vi "Get Tx Generic Raw Frame List.vi"(8 "error in":errorcluster, 11 "custom device ref in":T3 format="%.0x") -> (0 "error out":errorcluster, 2 "Raw Frame List":T1[](array[typedef]) {"Data" format="%.0x"; "HeaderInfo"."NetSelect" items=["FDX_TX_FRAME_DLY_A"=0, "FDX_TX_FRAME_DLY_B"=1, "FDX_TX_FRAME_BOTH "=3, "FDX_TX_FRAME_ONLY_A"=4, "FDX_TX_FRAME_ONLY_B "=5]; "HeaderInfo"."FrameStartMode" items=["FDX_TX_FRAME_START_IFG", "FDX_TX_FRAME_START_PGWT", "FDX_TX_FRAME_START_TRG"]; "HeaderInfo"."PhysErrorInjection" items=["FDX_TX_FRAME_ERR_OFF"=0, "FDX_TX_FRAME_ERR_CRC"=1, "FDX_TX_FRAME_ERR_ALI"=2, "FDX_TX_FRAME_ERR_PRE"=4, "FDX_TX_FRAME_ERR_PHY"=8]; "HeaderInfo"."SequenceNumberInit" items=["FDX_TX_FRAME_SEQ_INIT_AUTO"=65535]; "HeaderInfo"."SequenceNumberOffset" items=["FDX_TX_FRAME_SEQ_OFFS_AUTO "=65535]; "HeaderInfo"."PayloadGenerationMode" items=["FDX_TX_FRAME_PGM_USER"=0, "FDX_TX_FRAME_PGM_IP_PART"=1, "FDX_TX_FRAME_PGM_IP_FULL"=2, "FDX_TX_FRAME_PGM_IP_PART_TT"=10, "FDX_TX_FRAME_PGM_IP_FULL_TT"=20]; "HeaderInfo"."PayloadBufferMode" items=["FDX_TX_FRAME_PBM_STD", "FDX_TX_FRAME_PBM_MAC", "FDX_TX_FRAME_PBM_UDP"]}, 3 "custom device ref out":T3 format="%.0x", 4 "Found?":bool)   [LabVIEW 2020, in "AIM ARINC 664 Scripting.lvlib"]
uses:
  AIM ARINC 664 Scripting.lvlib
  <vilib>/NI VeriStand/Custom Device API/Custom Device Item Ref.ctl
  Shared/RawFrame.ctl
  <instrlib>/AIM GmbH/_AIM 664/_controls/queue_header_generic.ctl
  Constants.vi
  <vilib>/NI VeriStand/Custom Device Tools/Custom Device Utility Library/NI VeriStand - Search for Item by GUID.vi
  <vilib>/NI VeriStand/Custom Device API/Get Item Property (Variant).vi
  <vilib>/NI VeriStand/Custom Device API/Custom Device API.lvlib
  <vilib>/NI VeriStand/Custom Device Tools/Custom Device Utility Library/Custom Device Utility Library.lvlib
  <instrlib>/AIM GmbH/_AIM 664/AIM664LV.lvlib
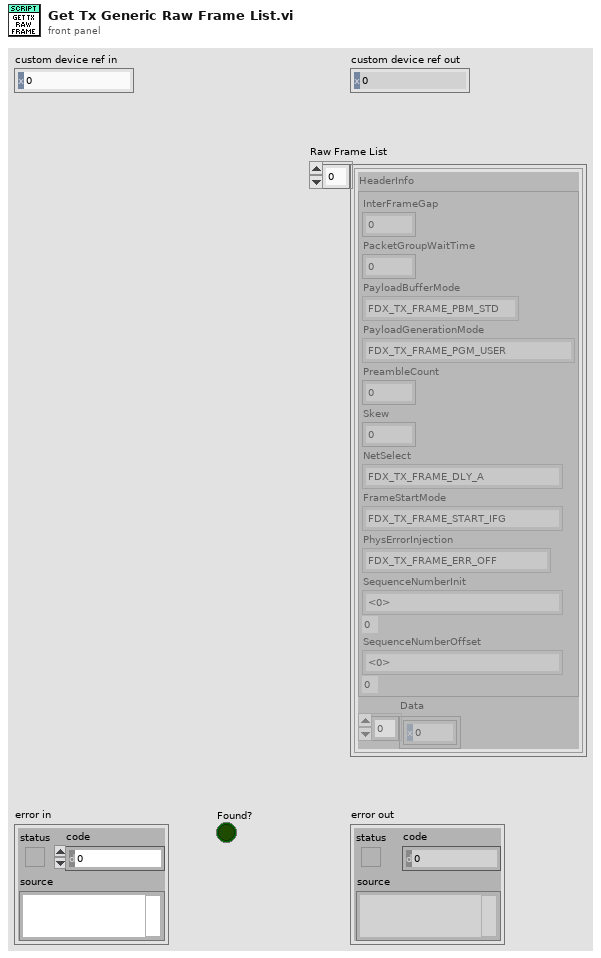
[diagram p1: front panel]
types:
  T1 = typedef "RawFrame.ctl" = cluster{"HeaderInfo":T2, "Data":u8[]}
  T2 = typedef "AIM664LV.lvlib/queue_header_generic.ctl" = cluster{"InterFrameGap":u32, "PacketGroupWaitTime":u32, "PayloadBufferMode":u8, "PayloadGenerationMode":u8, "PreambleCount":u8, "Skew":u32, "NetSelect":u8, "FrameStartMode":u8, "PhysErrorInjection":u32, "SequenceNumberInit":u16, "SequenceNumberOffset":u16}
  T3 = typedef "Custom Device API.lvlib/Custom Device Item Ref.ctl" = u64
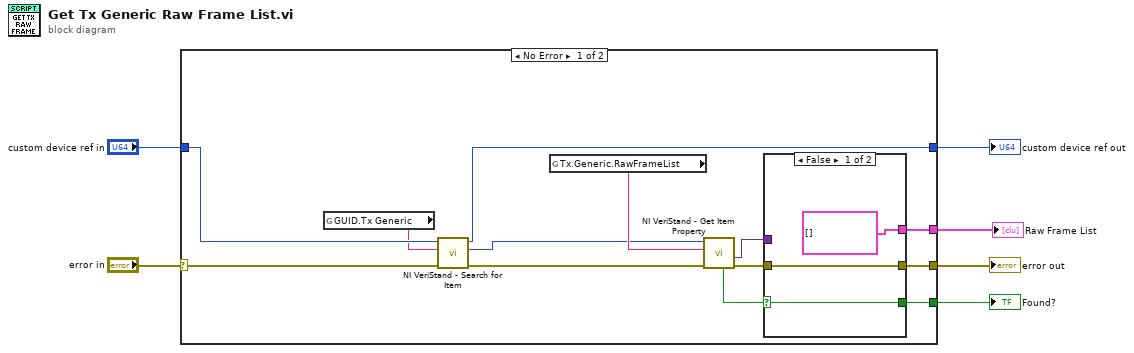
[diagram p0: block diagram]
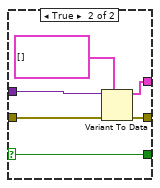
[diagram p2: hidden frame]
diagram:
  n1 = case shown="No Error" "error in" {
    selector: "error in" -> [w17 w30]
    tunnel: "custom device ref in" -> [w18 w29]
    tunnel: [w9 w30] -> w5
    tunnel: [w13 w29] -> w4
    tunnel: [w8 _] -> w1
    tunnel: [w11 _] -> w2
    frame No Error {
      n2 = global read "Constants.vi" "GUID.Tx Generic"() -> (w15:string)
      n3 = call-poly <vilib>:"NI VeriStand - Search for Item.vi"("error in"=w17, "Item GUID"=w15, "Section Ref in"=w18) -> ("error out"=w16:errorcluster, "Item Ref"=w14:T3, "Section Ref out"=w13:T3)  [unwired: 5 in, 1 out]
      n4 = global read "Constants.vi" "Tx.Generic.RawFrameList"() -> (w19:string)
      n5 = call-poly <vilib>:"NI VeriStand - Get Item Property.vi"("error in (no error)"=w16, "Property Name"=w19, "Item Ref in"=w14) -> ("error out"=w10:errorcluster, "Value"=w7:variant, "Found?"=w12:bool)  [unwired: 5 in, 1 out]
      n6 = case shown="False" w12 {
        selector: w12 -> [w21 w28]
        tunnel: [w21 w28] -> w11
        tunnel: w10 -> [w22 w27]
        tunnel: [w22 w23] -> w9
        tunnel: [T1[] [] ("Frame Array 2") w24] -> w8
        tunnel: w7 -> [_ w26]
        frame False {
        }
        frame True {
          n7 = Variant To Data(error in=w27, type=T1[] [] ("Frame Array 2"), Variant=w26) -> (data=w24:T1[], error out=w23:errorcluster)
        }
      }
    }
    frame Error {
    }
  }
  "error out" <- w5
  "custom device ref out" <- w4
  "Found?" <- w2
  "Raw Frame List" <- w1
